vi "Pre Launch Init.vi"(11 "Arduino_Stepper in":refnum<class "Arduino_Stepper.lvclass">) -> (0 "error out":errorcluster, 3 "Arduino_Stepper out":refnum<class "Arduino_Stepper.lvclass">)   [LabVIEW 2023, in "Arduino_TranslationStage_UI.lvlib" / "Arduino_Stepper.lvclass"]
doc: "(<B>Filename</B>: Actor Framework.lvlib:Actor.lvclass:Pre Launch Init.vi)\n\nDefines behavior that occurs after the Launch Nested Actor method is invoked but before the actor's Actor Core method begins running.\n\nBy default, this method does nothing. A descendant class may override it to define behavior."
uses:
  Arduino_Stepper.lvclass
  TranslationStage_UI/StageMoveDone_For_UI.ctl
  Arduino_Stepper.lvclass/Arduino_Stepper.ctl
  <vilib>/ActorFramework/Actor/Actor.lvclass
  typedefs/typedefs.lvlib
panel:
  in  "Variant":variant
  in  "Registers":u16[][](array[numeric])
  in  "Positions":T1={"CH1 Pos"=0.0, "CH2 Pos"=0.0, "CH3 Pos"=0.0, "CH4 Pos"=0.0, "Home?"=TRUE}
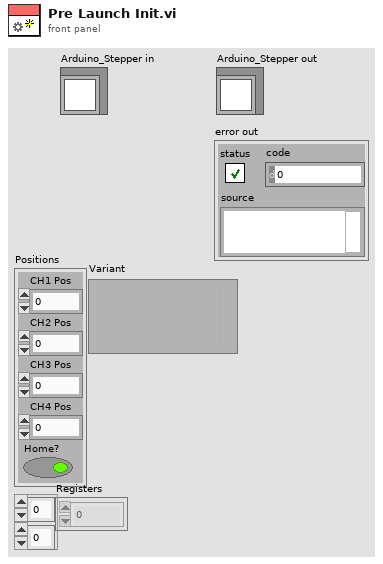
[diagram p1: front panel]
types:
  T1 = typedef "typedefs.lvlib/StageMoveDone_For_UI.ctl" = cluster{"CH1 Pos":sgl, "CH2 Pos":dbl, "CH3 Pos":dbl, "CH4 Pos":dbl, "Home?":bool}
  T2 = cluster{"Scanning Done":bool, "Axis":enum16{"X", "Y", "Z", "HOM"}}
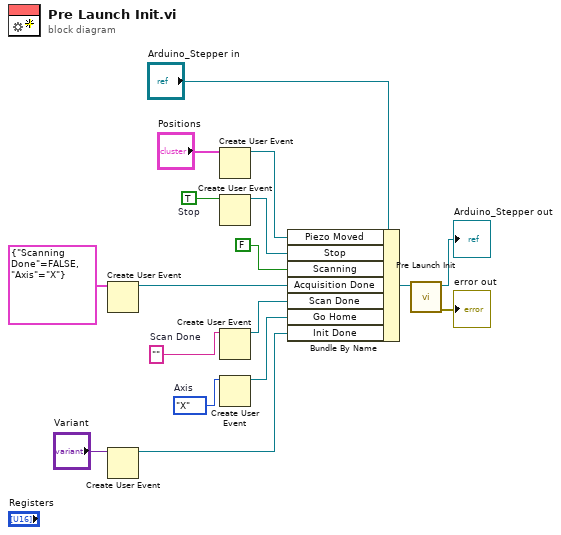
[diagram p0: block diagram]
diagram:
  w5 = enum16{"X", "Y", "Z", "HOM"}."X"  # Axis
  w11 = ""  # Scan Done
  w14 = TRUE  # Stop
  n1 = Create User Event(user event datatype=T2 {"Scanning Done"=FALSE, "Axis"=enum."X"} ("Acq Done Data")) -> (user event=w12:refnum<user-event>)  [unwired: 1 in, 1 out]
  n2 = Create User Event(user event datatype="Variant") -> (user event=w3:refnum<user-event>)  [unwired: 1 in, 1 out]
  n3 = Create User Event(user event datatype="Positions") -> (user event=w9:refnum<user-event>)  [unwired: 1 in, 1 out]
  n4 = Create User Event(user event datatype=w14) -> (user event=w15:refnum<user-event>)  [unwired: 1 in, 1 out]
  n5 = Create User Event(user event datatype=w11) -> (user event=w10:refnum<user-event>)  [unwired: 1 in, 1 out]
  n6 = Create User Event(user event datatype=w5) -> (user event=w6:refnum<user-event>)  [unwired: 1 in, 1 out]
  n7 = Bundle By Name(cluster="Arduino_Stepper in", "Piezo Moved"=w9, "Stop"=w15, "Scanning"=FALSE ("Cam Connected"), "Acquisition Done"=w12, "Scan Done"=w10, "Go Home"=w6, "Init Done"=w3) -> (w1:refnum<class "Arduino_Stepper.lvclass">)
  n8 = call-parent "Pre Launch Init.vi"("Actor in"=w1) -> ("error out"=→"error out":errorcluster, "Actor out"=→"Arduino_Stepper out":refnum<class "Arduino_Stepper.lvclass">)  [unwired: 9 in]
